vi "电话号码输入.vi"() -> ()   [LabVIEW 2018]
panel:
  in  "停止":bool
  in  "输入电话号码":string
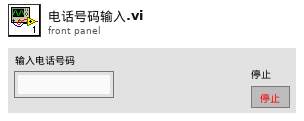
[diagram p1: front panel]
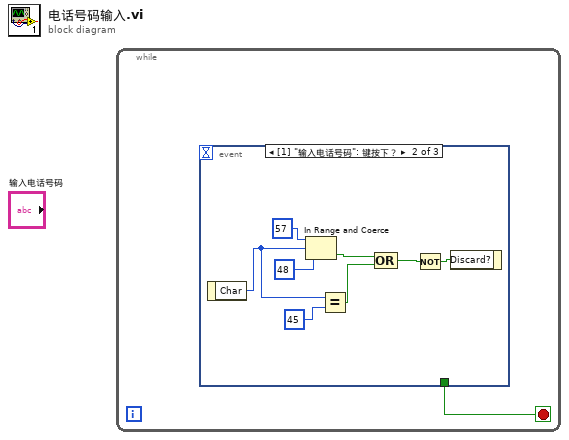
[diagram p0: block diagram]
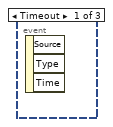
[diagram p2: hidden frame]
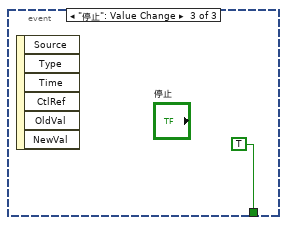
[diagram p3: hidden frame]
diagram:
  n1 = while {
    stop <- w1 stop-if-true
    n2 = event shown="[1] \"输入电话号码\": 键按下？" {
      selector: _ -> [_ _ _]
      dyn-events: _ -> [_ _ _]
      timeout: _ -> [_ _ _]
      tunnel: [_ _ TRUE] -> w1
      event Timeout {
        n3 = event-data() -> ()  [unwired: 1 in, 3 out]
      }
      event "输入电话号码": Key Down? {
        n4 = event-data() -> ("Char"=w7:i16)  [unwired: 1 in]
        n5 = In Range and Coerce(upper limit=i16 57 ("上限"), x=w7, lower limit=i16 48 ("下限")) -> (In Range?=w5:bool)  [unwired: 1 out]
        n6 = Equal?(x=w7, y=i16 45) -> (x = y?=w4:bool)
        n7 = Compound Arithmetic op=OR(w5, w4) -> (w3:bool)
        n8 = Not(x=w3) -> (.not. x?=w2:bool)
        n9 = event-data("Discard?"=w2) -> ()  [unwired: 1 in, 1 out]
      }
      event "停止": Value Change {
        n10 = event-data() -> ()  [unwired: 1 in, 6 out]
      }
    }
  }
